vi "sync and trig.vi"(8 "error in (no error)":errorcluster, 10 "time calibrate":dbl[](array[numeric]), 11 "USRP_1_x_200MHz in":refnum<class "USRP_1_x_200MHz.lvclass">) -> (0 "error out":errorcluster, 3 "USRP_1_x_200MHz out":refnum<class "USRP_1_x_200MHz.lvclass">)   [LabVIEW 2021, in "USRP_1_x_200MHz.lvclass"]
uses:
  USRP_1_x_200MHz.lvclass
  USRP_1_x_200MHz.lvclass/USRP_1_x_200MHz.ctl
  <vilib>/Utility/error.llb/Error Cluster From Error Code.vi
  <vilib>/rvi/errors/niLvFpgaAdjustHostInterfaceError.vi
  <vilib>/rvi/interface/nirviReadWriteControl/nirviReadWriteControl.xnode
  NiFpgaLv.dll
  <vilib>/rvi/interface/Simulation/niFpgaSimulationCallBeginRW.vi
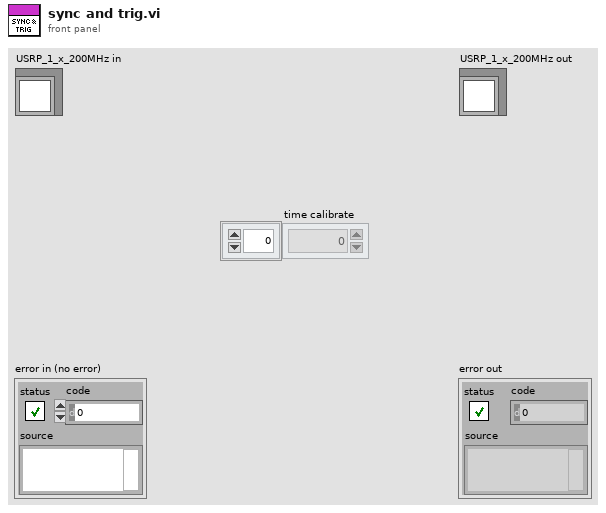
[diagram p1: front panel]
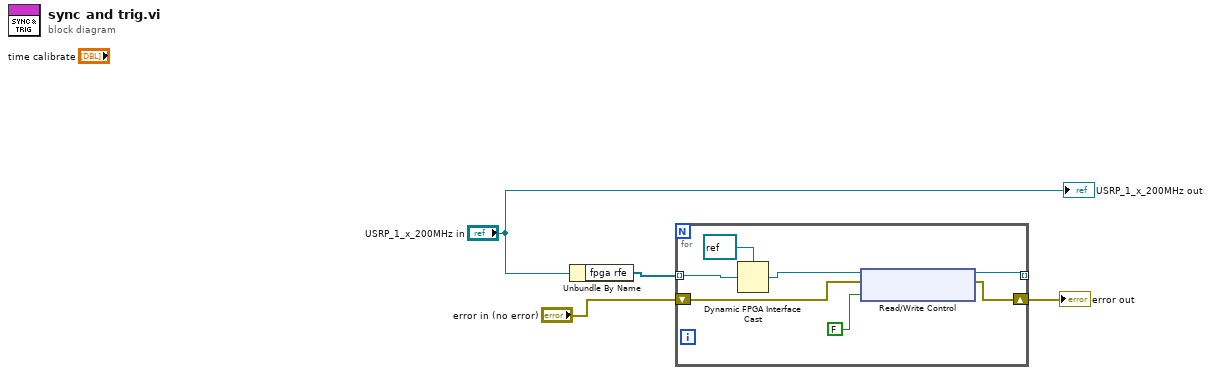
[diagram p0: block diagram]
diagram:
  n1 = Unbundle By Name("USRP_1_x_200MHz in") -> ("fpga rfe"=w4:refnum<k20>[])
  n2 = for {
    tunnel: w4 -> [w7] mode=indexing
    shift-right: [w8] -> w2
    shift-left: "error in (no error)" -> [w9]
    tunnel: [w11] -> _ mode=indexing
    n3 = Dynamic FPGA Interface Cast(Session In=refnum<k20> refnum ("FPGA VI Reference Out"), Type=w7) -> (Session Out=w6:refnum<k20>)
    n4 = xnode "Read/Write Control"("FPGA VI Reference In"=w6, "error in"=w9, "reset system clock"=FALSE) -> ("FPGA VI Reference Out"=w11:refnum<k20>, "error out"=w8:errorcluster)
  }
  "error out" <- w2
  "USRP_1_x_200MHz out" <- "USRP_1_x_200MHz in"
